vi "Abort notifier.vi"(4 "error in (no error)":errorcluster) -> (0 "error out":errorcluster, 2 "x > 0?":bool)   [LabVIEW 2020]
doc: "Sends <B>Abort</B> notifier to terminate DAQ thread."
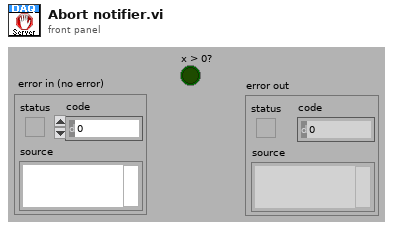
[diagram p1: front panel]
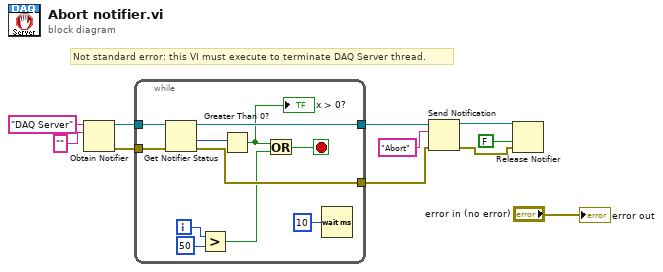
[diagram p0: block diagram]
diagram:
  # "Not standard error: this VI must execute to terminate DAQ Server thread."
  n1 = Obtain Notifier(name (unnamed)="DAQ Server", notification data type="") -> (notifier out=w5:refnum<notifier>, error out=w4:errorcluster)  [unwired: 2 in, 1 out]
  n2 = while {
    tunnel: w5 -> [w21]
    tunnel: w4 -> [w16]
    tunnel: [w19] -> w3
    tunnel: [w18] -> w2
    i -> [w14]
    stop <- w15 stop-if-true
    n3 = Get Notifier Status(notifier=w21, error in (no error)=w16) -> (notifier out=w19:refnum<notifier>, # waiting=w20:i32, error out=w18:errorcluster)  [unwired: 2 out]
    n4 = Greater?(x=w14, y=50) -> (0:w12:bool)
    n5 = Greater Than 0?(x=w20) -> (x > 0?=w17:bool)
    "x > 0?" <- w17
    n6 = Or(x=w17, y=w12) -> (x .or. y?=w15:bool)
    n7 = Wait (ms)(milliseconds to wait=10) -> ()  [unwired: 1 out]
  }
  n8 = Send Notification(notification="Abort", notifier=w3, error in (no error)=w2) -> (notifier out=w10:refnum<notifier>, error out=w9:errorcluster)
  n9 = Release Notifier(notifier=w10, force destroy? (F)=FALSE, error in (no error)=w9) -> ()  [unwired: 3 out]
  "error out" <- "error in (no error)"
